vi "Dialog.vi"(8 "Error in":errorcluster caption="Error in (no error)", 10 "message":string="Click OK to release mask.") -> (0 "Error out":errorcluster)   [LabVIEW 2016, in "Rectangle Mask.lvclass"]
uses:
  Rectangle Mask.lvclass
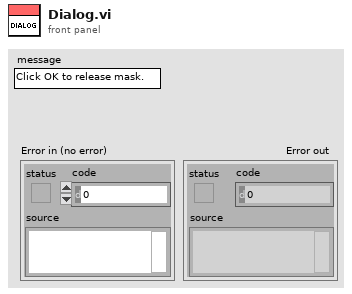
[diagram p1: front panel]
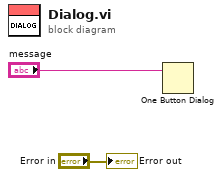
[diagram p0: block diagram]
diagram:
  n1 = One Button Dialog(message="message") -> ()  [unwired: 1 in, 1 out]
  "Error out" <- "Error in"
